vi "PID Rotation control.vi"(6 "Gyro Rate":dbl, 7 "PID gains":T1={"proportional gain (Kc)"=2.0, "integral time (Ti, min)"=0.1, "derivative time (Td, min)"=0.0} {"derivative time (Td, min)" format="%.3f"; "integral time (Ti, min)" format="%.3f"; "proportional gain (Kc)" format="%.3f"}, 9 "Gyro":dbl, 10 "PID gains 2":T1={"proportional gain (Kc)"=0.030222000000000006, "integral time (Ti, min)"=0.025000000000000015, "derivative time (Td, min)"=0.0} {"derivative time (Td, min)" format="%.3f"; "integral time (Ti, min)" format="%.3f"; "proportional gain (Kc)" format="%.3f"}, 11 "Numeric":dbl) -> (3 "output":dbl)   [LabVIEW 2014]
uses:
  <vilib>/addons/control/pid/pid.llb/PID (DBL).vi
  <vilib>/addons/control/pid/NI_PID_pid.lvlib
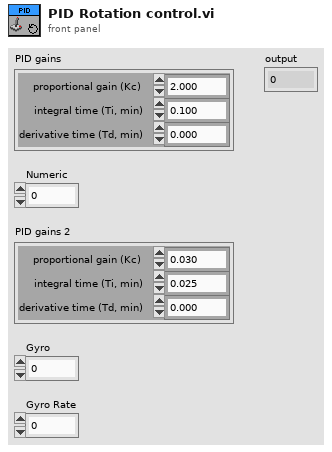
[diagram p1: front panel]
types:
  T1 = cluster{"proportional gain (Kc)":dbl, "integral time (Ti, min)":dbl, "derivative time (Td, min)":dbl}
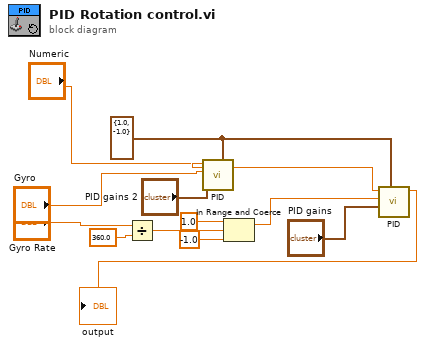
[diagram p0: block diagram]
diagram:
  w13 = cluster{"output high":dbl, "output low":dbl} {"output high"=1.0, "output low"=-1.0} ("output range")
  n1 = Divide(x="Gyro Rate", y=360.0) -> (x/y=w7:dbl)
  n2 = call-poly <vilib>:"PID.vi"("output range"=w13, "PID gains"="PID gains 2", "process variable"="Gyro", "setpoint"="Numeric") -> ("output"=w12:dbl)  [unwired: 6 in, 1 out]
  n3 = In Range and Coerce(upper limit=1.0, x=w7, lower limit=-1.0) -> (coerced(x)=w8:dbl)  [unwired: 1 out]
  n4 = call-poly <vilib>:"PID.vi"("output range"=w13, "PID gains"="PID gains", "process variable"=w8, "setpoint"=w12) -> ("output"=→"output":dbl)  [unwired: 6 in, 1 out]
